vi "Initiate.vi"(8 "error in (no error)":errorcluster, 10 "initiate mode (0:continuous)":u16(ring) items=["Continuous Initiate", "Single Initiate", "Stop Continuous"], 11 "VISA resource name":refnum<visa-resource-name>) -> (0 "error out":errorcluster, 3 "VISA resource name out":refnum<visa-resource-name>)   [LabVIEW 2016, in "Agilent 4263X.lvlib"]
doc: "This VI causes all sequences to exit the idle state and enter the initiate state. This VI causes the trigger system to initiate and complete one full trigger cycle, returning to the idle state on completion.\n\nNOTE: If the instrument is not in the idle state upon execution, then this VI has no effect on the current state of the instrument and an error will be generated by the instrument and can be read by the Error Query VI."
uses:
  <instrlib>/Agilent 4263X/Agilent 4263X.lvlib
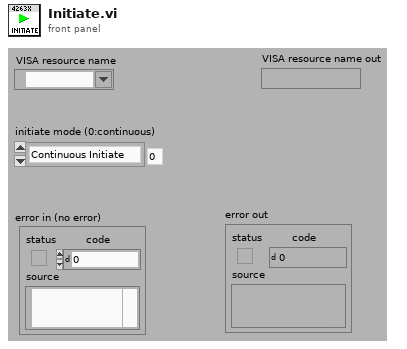
[diagram p1: front panel]
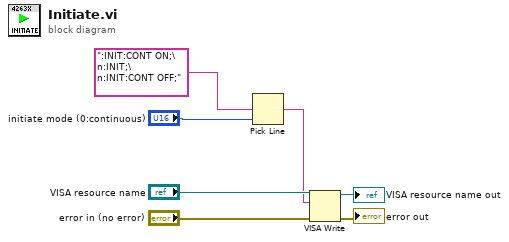
[diagram p0: block diagram]
diagram:
  n1 = Pick Line(multi-line string=":INIT:CONT ON;\n:INIT;\n:INIT:CONT OFF;", line index="initiate mode (0:continuous)") -> (output string=w1:string)  [unwired: 1 in]
  n2 = VISA Write(VISA resource name="VISA resource name", write buffer=w1, error in (no error)="error in (no error)") -> (VISA resource name out=→"VISA resource name out":refnum<visa-resource-name>, error out=→"error out":errorcluster)  [unwired: 1 out]
